vi "Remove Line From File.vi"(7 "Check Only? (f)":bool, 8 "Error In":errorcluster, 9 "Line":string="i2c-bcm2708", 10 "File Path":string="cat /etc/modules", 11 "Install LV Data":T1={"SSH Session"=refnum, "Status Log"="", "Detailed Log"="", "Credentials"={"Hostname or IP"="192.168.7.2", "Username"="root", "Password"=""}, "Target Info"={"OS Version"="", "CPU"="", "Systemd Version"="", "Internet Access"=FALSE, "Device Type"=""}, "Reboot Required?"=FALSE}) -> (0 "Error Out":errorcluster, 1 "Log":string, 2 "Line Previously Present?":bool, 3 "Install LV Data":T1={"SSH Session"=refnum, "Status Log"="", "Detailed Log"="", "Credentials"={"Hostname or IP"="192.168.7.2", "Username"="root", "Password"=""}, "Target Info"={"OS Version"="", "CPU"="", "Systemd Version"="", "Internet Access"=FALSE, "Device Type"=""}, "Reboot Required?"=FALSE})   [LabVIEW 2014, in "LMH-LINX.lvlib"]
uses:
  LMH-LINX.lvlib
  Install LV Data.ctl
  C:/github/makerhub/LINX/LabVIEW/vi.lib/MakerHub/LINX/Resources/Renci.SshNet.dll
  Resources/Renci.SshNet.dll
  Target Info.ctl
  <vilib>/regexp/Match Regular Expression.xnode
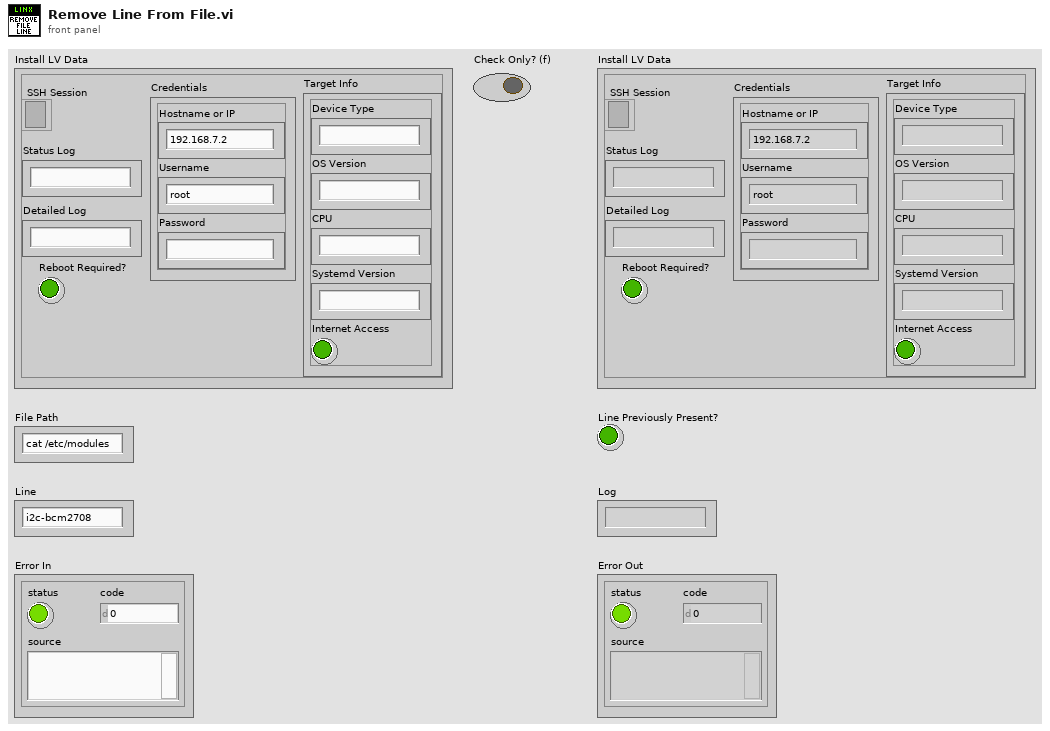
[diagram p1: front panel]
types:
  T1 = typedef "LMH-LINX.lvlib/Install LV Data.ctl" = cluster{"SSH Session":refnum<k24>, "Status Log":string, "Detailed Log":string, "Credentials":cluster{"Hostname or IP":string, "Username":string, "Password":string}, "Target Info":T2, "Reboot Required?":bool}
  T2 = typedef "LMH-LINX.lvlib/Target Info.ctl" = cluster{"OS Version":string, "CPU":string, "Systemd Version":string, "Internet Access":bool, "Device Type":string}
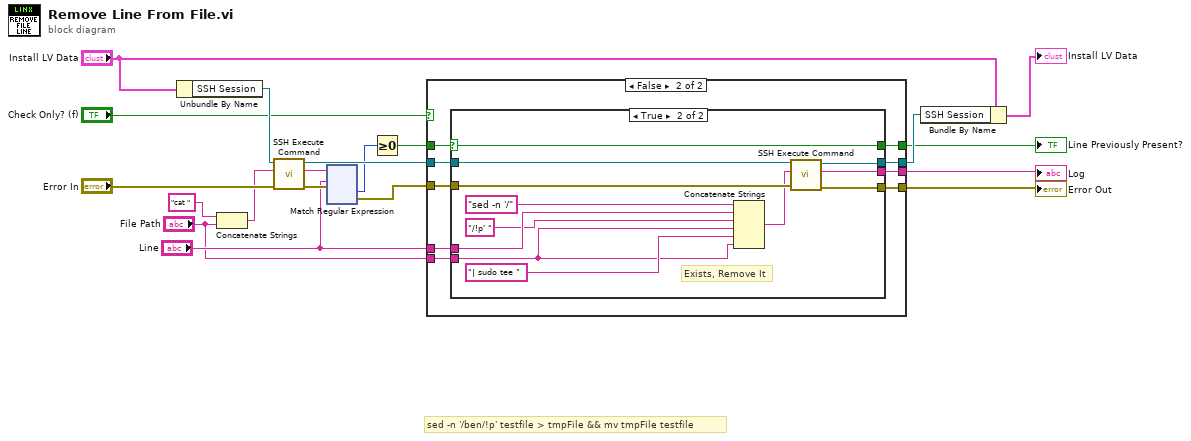
[diagram p0: block diagram]
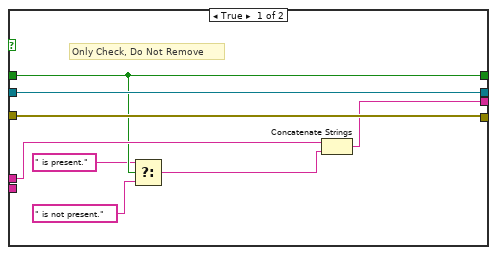
[diagram p2: hidden frame]
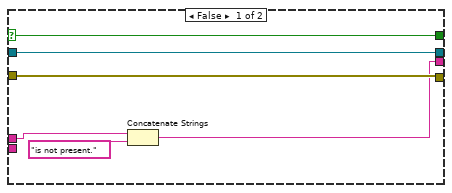
[diagram p3: hidden frame]
diagram:
  # "sed -n '/ben/!p' testfile > tmpFile && mv tmpFile testfile"
  n1 = Unbundle By Name("Install LV Data") -> ("SSH Session"=w17:refnum<k24>)
  n2 = Concatenate Strings("cat " ("string"), "File Path") -> (w8:string)
  n3 = call "SSH Execute Command.vi"("Error In"="Error In", "Command"=w8, "SSH Session"=w17) -> ("Error Out"=w14:errorcluster, "Std Out"=w10:string, "SSH Session"=w15:refnum<k24>)  [unwired: 6 in]
  n4 = xnode "Match Regular Expression"("input string"=w10, "regular expression"="Line", "error in"=w14) -> ("offset past match"=w12:i32, "error out"=w13:errorcluster)  [unwired: 3 in, 3 out]
  n5 = Greater Or Equal To 0?(x=w12) -> (x >= 0?=w11:bool)
  n6 = case shown="False" "Check Only? (f)" {
    tunnel: w15 -> [w27 w36]
    tunnel: w13 -> [w26 w35]
    tunnel: w11 -> [w23 w34]
    tunnel: "Line" -> [w24 w33]
    tunnel: [w26 w32] -> w6
    tunnel: [w25 w31] -> w5
    tunnel: [w27 w30] -> w4
    tunnel: "File Path" -> [_ w29]
    tunnel: [w23 w28] -> w1
    frame True {
      # "Only Check, Do Not Remove"
      n7 = Select(t=" is present.", s=w23, f=" is not present.") -> (s? t:f=w20:string)
      n8 = Concatenate Strings(w24, w20) -> (w25:string)
    }
    frame False {
      n9 = case shown="True" w34 {
        selector: w34 -> [w40 w49]
        tunnel: [w37 w43] -> w31
        tunnel: [w42 w54] -> w32
        tunnel: [w41 w53] -> w30
        tunnel: w36 -> [w41 w52]
        tunnel: w35 -> [w42 w51]
        tunnel: w33 -> [w39 w47]
        tunnel: w29 -> [_ w44]
        tunnel: [w40 w49] -> w28
        frame False {
          n10 = Concatenate Strings(w39, "is not present." ("string")) -> (w37:string)
        }
        frame True {
          # "Exists, Remove It"
          n11 = Concatenate Strings("sed -n '/", w47, "/!p' ", w44, "| sudo tee ", w44) -> (w50:string)
          n12 = call "SSH Execute Command.vi"("Error In"=w51, "Command"=w50, "SSH Session"=w52) -> ("Error Out"=w54:errorcluster, "Std Out"=w43:string, "SSH Session"=w53:refnum<k24>)  [unwired: 6 in]
        }
      }
    }
  }
  "Log" <- w5
  "Error Out" <- w6
  "Line Previously Present?" <- w1
  n13 = Bundle By Name(cluster="Install LV Data", "SSH Session"=w4) -> (→"Install LV Data":T1)
